vi "Panel.vi"() -> ()   [LabVIEW 2014]
uses:
  ISCO3.LLB/Pump start time.glb
  CONTROL.LLB/Remote/local.vi
panel:
  in  "btnExit":bool
  in  "?":bool
  out "TOTAL TIME, ms":u32
  in  "SAMPLE TIME, ms":u32=500
  out "Pump status.":T1(array[cluster])
  out "Multipump data.":T2 {"Total volume (liters)." format="%.5e"; "Pressure (psi)." format="%.5e"; "Flow rate (liters/min)." format="%.5e"}
  out "Digital input string.":string
  out "Analog input Voltages.":T3 {"ANLG5 = pin 2 , P107 auxiliary DB25 connector." format="%.2f"; "ANLG4 = analog input 1 of the accessory connector." format="%.2f"; "ANLG3 = analog input 2 of the accessory connector." format="%.2f"; "ANLG2 = pin 15 , P107 auxiliary DB25 connector and analog input 3 of the accessory connector." format="%.2f"; "ANLG1 = pin 21, P114." format="%.2f"}
  in  "Tasks.":T4
  in  "Remote/Local/External (0:Remote).":enum16{"REMOTE", "LOCAL", "EXTERNAL"}(ring)
  out "Pump C output.":T5={"Flow Rate A"=2.5, "FS Units A"=0, "Pressure A"=0.0, "PS Units A"=0, "Volume Remaining  C"=507.38, "Vol Units A"=0, "Status A"="STOPPED REMOTE  ", "Run time (Hr:Min:sec) A"=""} {"Vol Units A" items=["ml"]; "PS Units A" items=["psi", "atm", "bar", "kpa"]; "FS Units A" items=["ml/min", "ml/hr", "ul/min", "ul/hr"]; "Pressure A" format="%.2f"; "Flow Rate A" format="%.4f"; "Volume Remaining  C" scale=0.0..-1.0 scale format="%.1f"}
  out "Pump C Model":string="MODEL 500D PUMP; REV=G"
  in  "Pump C Settings":T6={"Mode A"=0, "Flow Setpoint A"=2.5, "FS Units A"=0, "Pressure Setpoint A"=100.0, "PS Units A"=0, "Refill Rate A"=204.0, "F=STOP/T=RUN"=FALSE} {"PS Units A" items=["psi", "atm", "bar", "kpa"]; "Refill Rate A" format="%.4f"; "Pressure Setpoint A" format="%.2f"; "FS Units A" items=["ml/min", "ml/hr", "ul/min", "ul/hr"]; "Flow Setpoint A" format="%.4f"; "Mode A" items=["Constant Flow", "Constant Pressure", "Refill", "Rapid Pressurization", "Single Pump Press Gradient", "Single Pump FR Gradient"]}
  out "Pump B output.":T7={"Flow Rate A"=15.0, "FS Units A"=0, "Pressure A"=0.0, "PS Units A"=0, "Volume Remaining  B"=94.65678, "Vol Units A"=0, "Status A"="STOPPED REMOTE  ", "Run time (Hr:Min:sec) A"=""} {"Vol Units A" items=["ml"]; "PS Units A" items=["psi", "atm", "bar", "kpa"]; "FS Units A" items=["ml/min", "ml/hr", "ul/min", "ul/hr"]; "Pressure A" format="%.2f"; "Flow Rate A" format="%.4f"; "Volume Remaining  B" scale format="%.1f"}
  out "Pump B Model":string="MODEL 100DM PUMP; REV=G"
  in  "Pump B Settings":T6={"Mode A"=0, "Flow Setpoint A"=15.0, "FS Units A"=0, "Pressure Setpoint A"=100.0, "PS Units A"=0, "Refill Rate A"=30.0, "F=STOP/T=RUN"=FALSE} {"PS Units A" items=["psi", "atm", "bar", "kpa"]; "Refill Rate A" format="%.4f"; "Pressure Setpoint A" format="%.2f"; "FS Units A" items=["ml/min", "ml/hr", "ul/min", "ul/hr"]; "Flow Setpoint A" format="%.4f"; "Mode A" items=["Constant Flow", "Constant Pressure", "Refill", "Rapid Pressurization", "Single Pump Press Gradient", "Single Pump FR Gradient"]}
  out "Pump A output.":T8={"Flow Rate A"=120.0, "FS Units A"=0, "Pressure A"=0.0, "PS Units A"=0, "Volume Remaining  A"=372.35144, "Vol Units A"=0, "Status A"="STOPPED REMOTE  ", "Run time (Hr:Min:sec) A"=""} {"Vol Units A" items=["ml"]; "PS Units A" items=["psi", "atm", "bar", "kpa"]; "FS Units A" items=["ml/min", "ml/hr", "ul/min", "ul/hr"]; "Pressure A" format="%.2f"; "Flow Rate A" format="%.4f"; "Volume Remaining  A" scale format="%.1f"}
  out "Pump A Model":string="MODEL 500D PUMP; REV=G"
  in  "Pump A Settings":T6={"Mode A"=0, "Flow Setpoint A"=120.0, "FS Units A"=0, "Pressure Setpoint A"=100.0, "PS Units A"=0, "Refill Rate A"=204.0, "F=STOP/T=RUN"=FALSE} {"PS Units A" items=["psi", "atm", "bar", "kpa"]; "Refill Rate A" format="%.4f"; "Pressure Setpoint A" format="%.2f"; "FS Units A" items=["ml/min", "ml/hr", "ul/min", "ul/hr"]; "Flow Setpoint A" format="%.4f"; "Mode A" items=["Constant Flow", "Constant Pressure", "Refill", "Rapid Pressurization", "Single Pump Press Gradient", "Single Pump FR Gradient"]}
  in  "Control mode (0:INDEPENDENT).":T9(ring)
  # "Status"
  # "Pump Model"
  # "Mode"
  # "Flow  Rate Setpt"
  # "Pressure Setpt"
  # "Refill Rate Setpt"
  # "STOP/RUN"
  # "C"
  # "Volume Remaining"
  # "Run Duration"
  # "B"
  # "Volume Remaining"
  # "Run Duration"
  # "A"
  # "Volume Remaining"
  # "Run Duration"
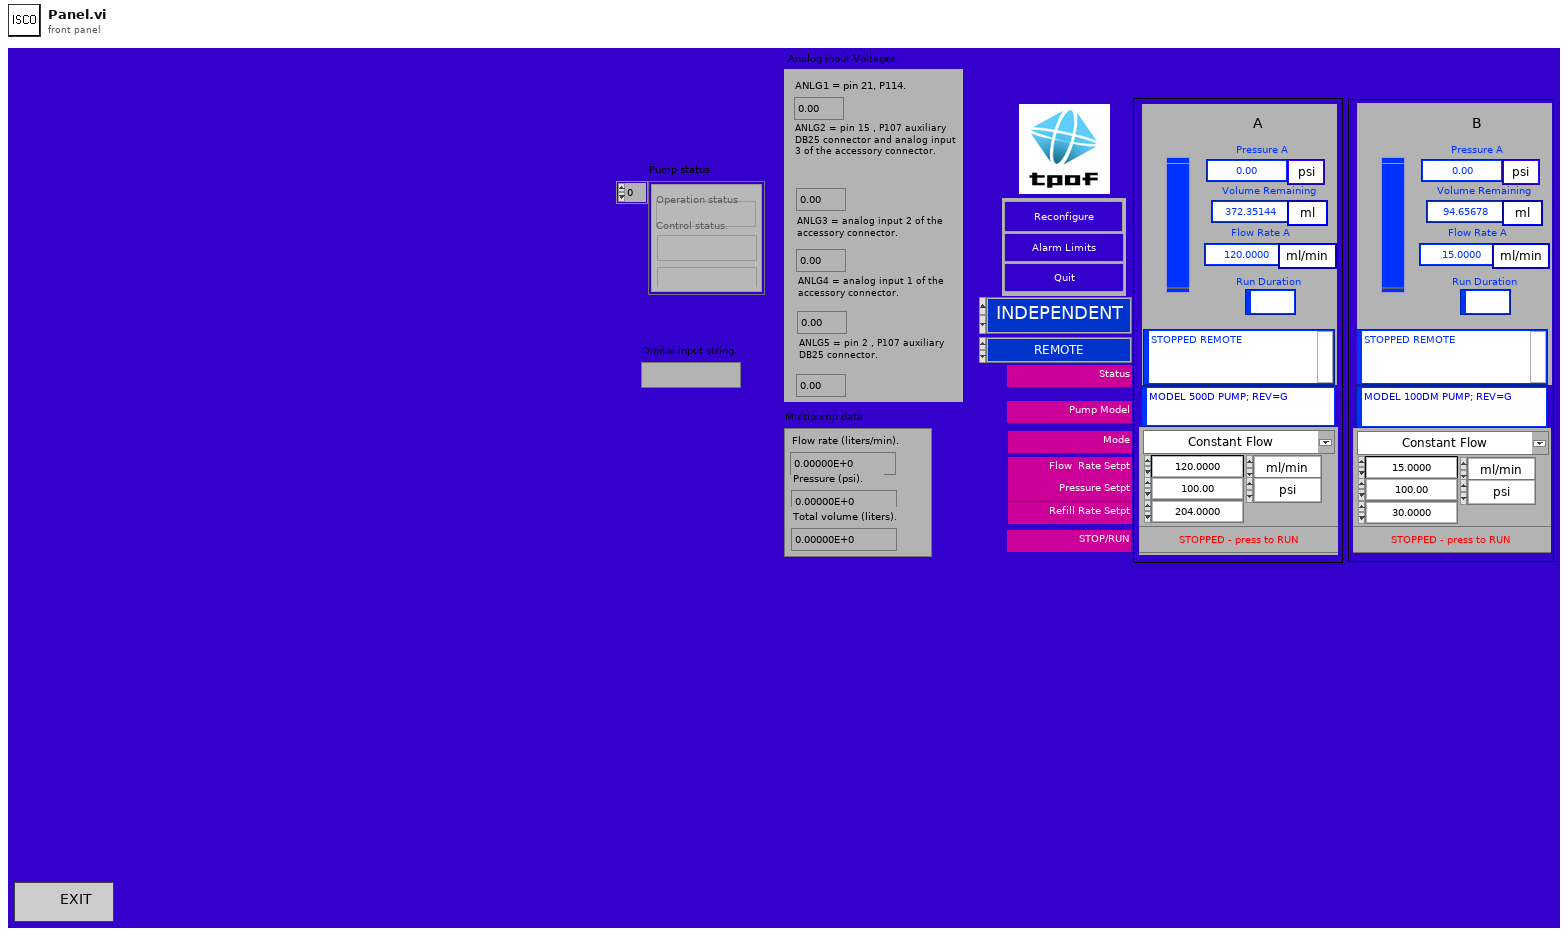
[diagram p1: front panel]
types:
  T1 = cluster{"Operation status":string, "Control status.  ":string, "Problem status.  ":string}[]
  T2 = cluster{"Flow rate (liters/min).  ":dbl, "Pressure (psi).  ":dbl, "Total volume (liters).  ":dbl}
  T3 = cluster{"ANLG1 = pin 21, P114.  ":dbl, "ANLG2 = pin 15 , P107 auxiliary DB25 connector and analog input 3 of the accessory connector.  ":dbl, "ANLG3 = analog input 2 of the accessory connector.  ":dbl, "ANLG4 = analog input 1 of the accessory connector.  ":dbl, "ANLG5 = pin 2 , P107 auxiliary DB25 connector.  ":dbl}
  T4 = cluster{"Reconfigure":bool, "Alarm Limits":bool, "Quit":bool}
  T5 = cluster{"Flow Rate A":sgl, "FS Units A":u16, "Pressure A":sgl, "PS Units A":u16, "Volume Remaining  C":sgl, "Vol Units A":u16, "Status A":string, "Run time (Hr:Min:sec) A":string}
  T6 = cluster{"Mode A":u16, "Flow Setpoint A":sgl, "FS Units A":u16, "Pressure Setpoint A":sgl, "PS Units A":u16, "Refill Rate A":sgl, "F=STOP/T=RUN":bool}
  T7 = cluster{"Flow Rate A":sgl, "FS Units A":u16, "Pressure A":sgl, "PS Units A":u16, "Volume Remaining  B":sgl, "Vol Units A":u16, "Status A":string, "Run time (Hr:Min:sec) A":string}
  T8 = cluster{"Flow Rate A":sgl, "FS Units A":u16, "Pressure A":sgl, "PS Units A":u16, "Volume Remaining  A":sgl, "Vol Units A":u16, "Status A":string, "Run time (Hr:Min:sec) A":string}
  T9 = enum16{"INDEPENDENT", "CONTIN CONST FLOW", "CONTIN CONST PRESS", "MODIFIER"}
  T10 = cluster{"Serial port":i32, "Baud rate":u16, "Controller":i32}
  T11 = cluster{"Mode A":u16, "Flow Setpoint A":sgl, "FS Units A":u16, "Pressure Setpoint A":sgl, "PS Units A":u16, "Refill Rate A":sgl, "F=STOP/T=RUN":bool}[]
  T12 = cluster{"Pump A.  ":string, "Pump B.  ":string, "Pump C.  ":string}
  T13 = cluster{"Maximum pressure (current units). ":sgl, "Maximum flow rate (current units).  ":sgl, "Maximum refill rate (currents units).  ":sgl, "Maximum volume (milliliters).  ":sgl}
  T14 = cluster{"Maximum pressure ":sgl, "Maximum flow rate.  ":sgl, "Maximum refill rate.  ":sgl, "Maximum volume.  ":sgl}
  T15 = cluster{"Maximum pressure setpoint.  ":sgl, "Minimum pressure setpoint":sgl, "Maximum flow rate.  ":sgl, "Minimum flow rate.  ":sgl, "Maximum flow rate in constant pressure mode.  ":sgl}
  T16 = cluster{"Maximum pressure setpoint (psi).  ":sgl, "Minimum pressure setpoint (psi).  ":sgl, "Maximum flow rate (liters/minute).  ":sgl, "Minimum flow rate (liters/minute).  ":sgl, "Maximum flow rate in constant pressure mode (liters/minute).  ":sgl}
  T17 = cluster{cluster{"Maximum pressure ":sgl, "Maximum flow rate.  ":sgl, "Maximum refill rate.  ":sgl, "Maximum volume.  ":sgl}[], cluster{"Maximum pressure setpoint (psi).  ":sgl, "Minimum pressure setpoint (psi).  ":sgl, "Maximum flow rate (liters/minute).  ":sgl, "Minimum flow rate (liters/minute).  ":sgl, "Maximum flow rate in constant pressure mode (liters/minute).  ":sgl}[]}
  T18 = enum32{"No op", "Reconfigure", "alarm limits", "Quit"}
  T19 = cluster{"Duration of run - pump A\n(Hours:minutes:seconds":string, "Duration of run - pump B\n(Hours:minutes:seconds":string, "Duration of run - pump C\n(Hours:minutes:seconds":string}
  T20 = cluster{"Time limit exceeded?  ":bool, "Bad checksum?":bool, "Busy?":bool}
  T21 = cluster{"Flow rate.  ":sgl, "Pressure.  ":sgl, "Volume remaining.  ":sgl, "Operation status.  ":string, "Control status.  ":string, "Problem status.  ":string}[]
  T22 = cluster{"ANLG1 = pin 21, P114.  ":dbl, "ANLG2 = pin 15 , P107 auxiliary DB25 connector and analog input 2 of the accessory connector.  ":dbl, "ANLG3 = analog input 2 of the accessory connector.  ":dbl, "ANLG4 = analog input 1 of the accessory connector.  ":dbl, "ANLG5 = pin 2 , P107 auxiliary DB25 connector.  ":dbl}
  T23 = cluster{"Maximum pressure setpoint (psi).  ":sgl, "Minimum pressure setpoint (psi).  ":sgl, "Maximum flow rate (liters/minute).  ":sgl, "Minimum flow rate (liters/minute).  ":sgl, "Maximum flow rate in constant pressure mode (liters/minute).  ":sgl}[]
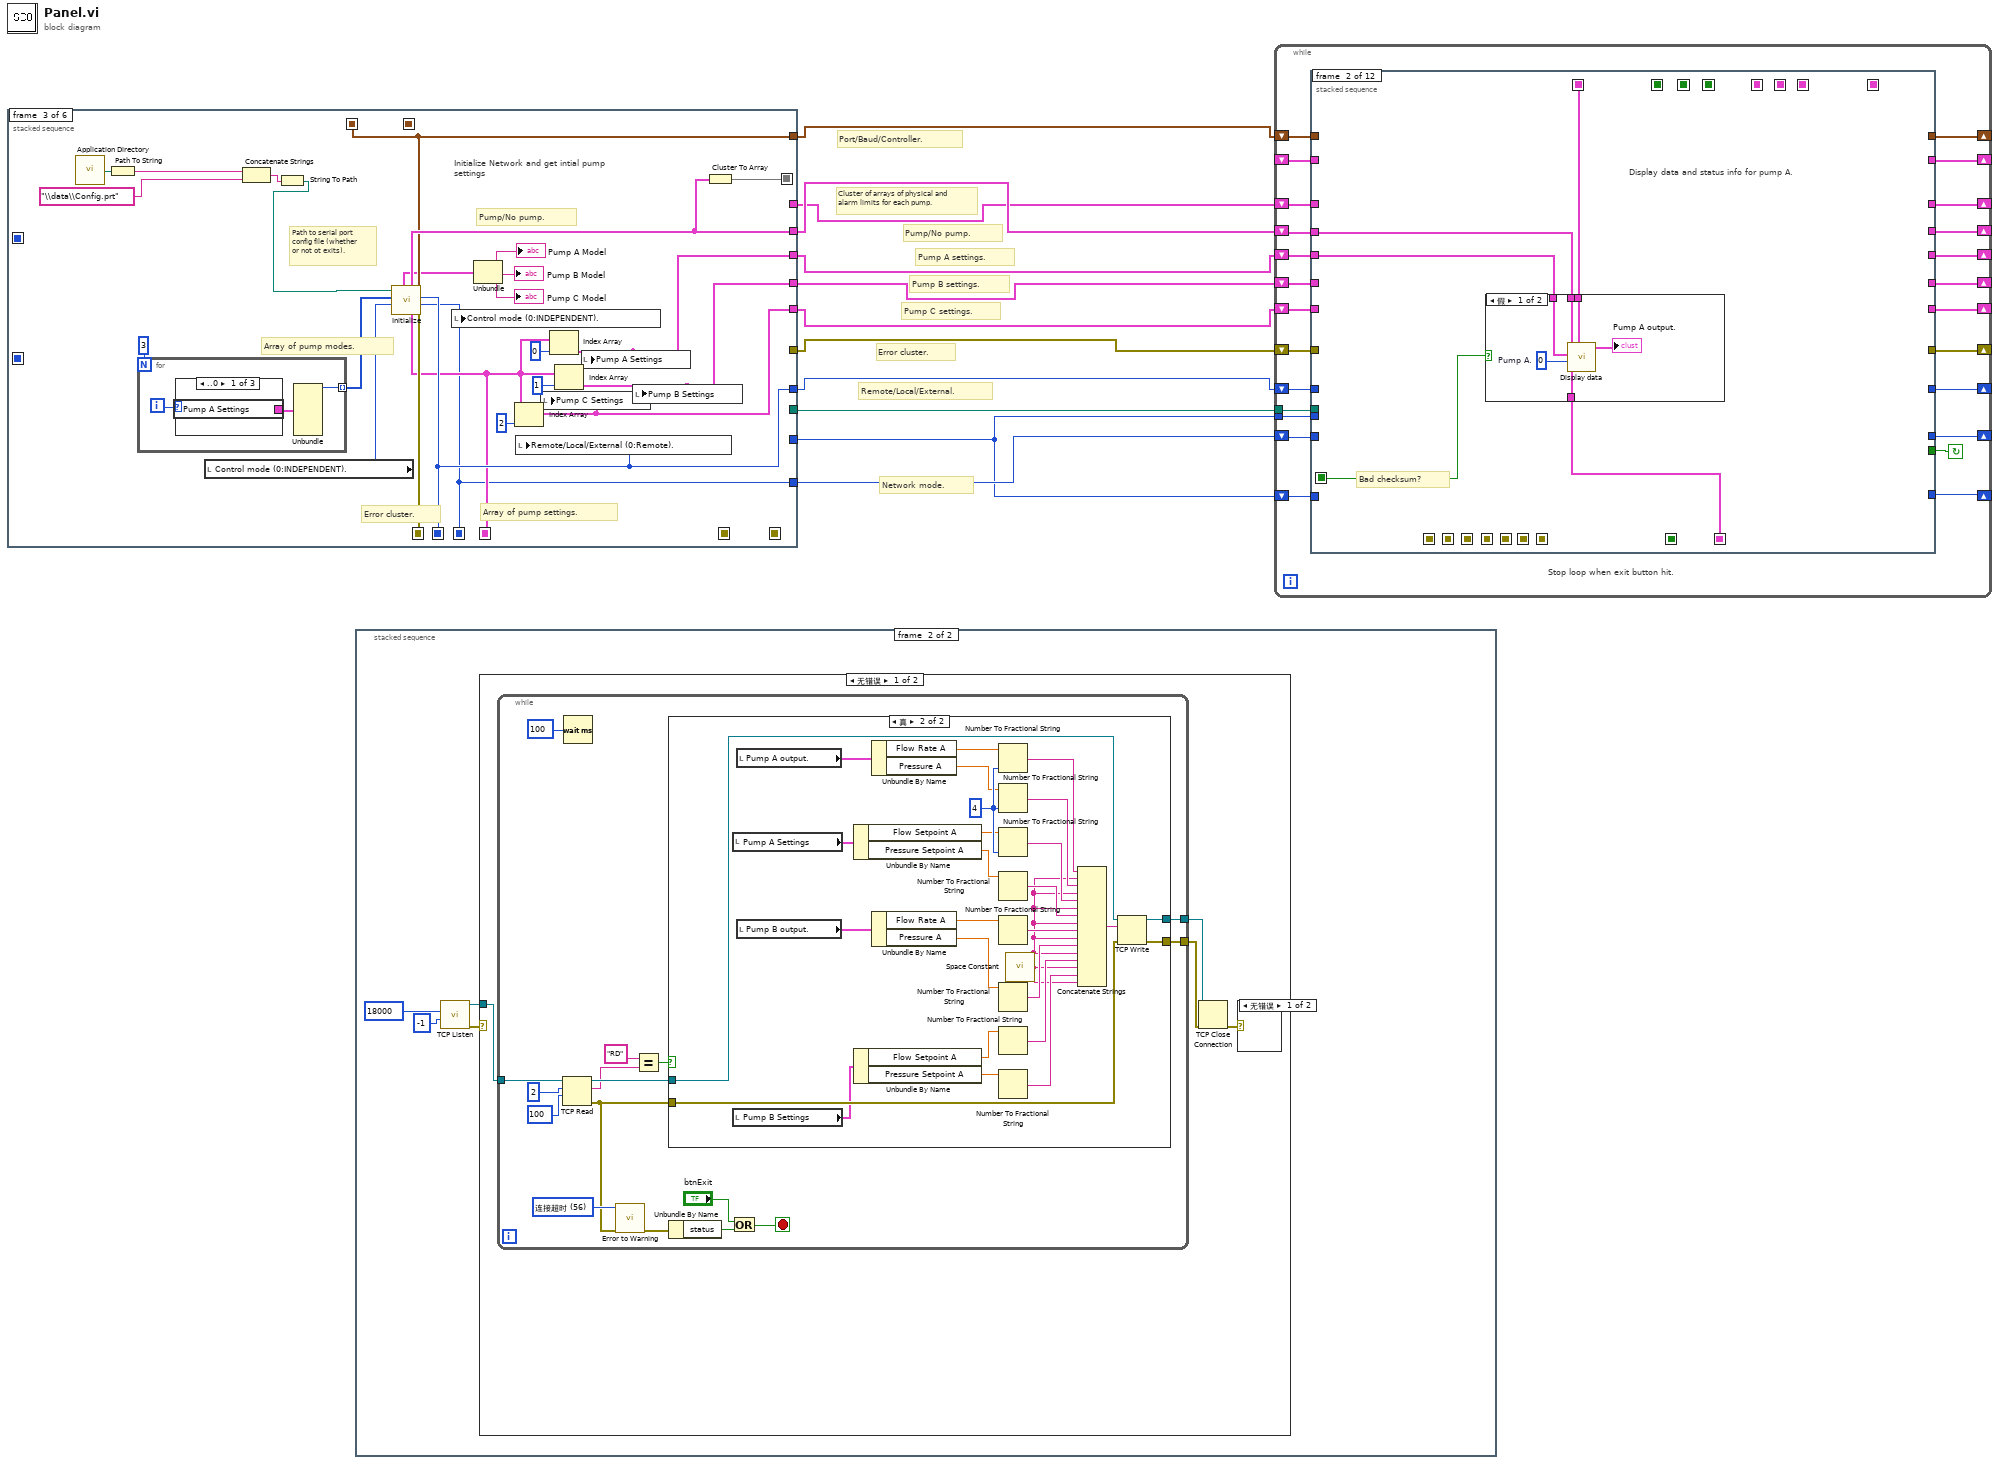
[diagram p0: block diagram]
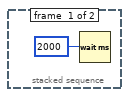
[diagram p2: hidden frame]
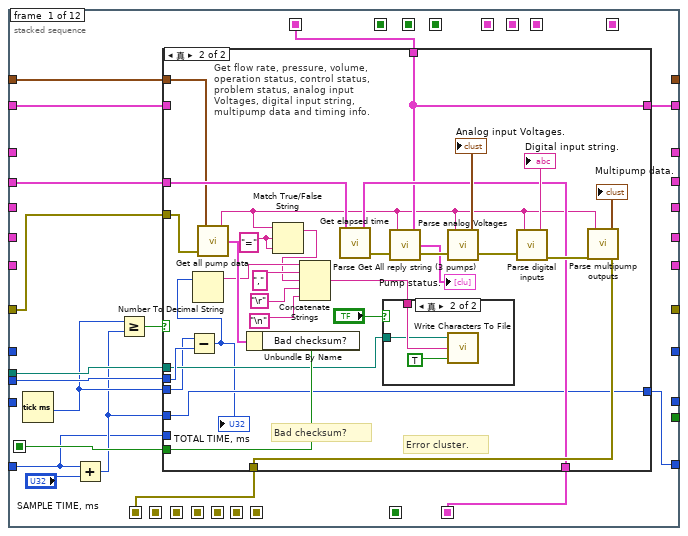
[diagram p6: hidden frame]
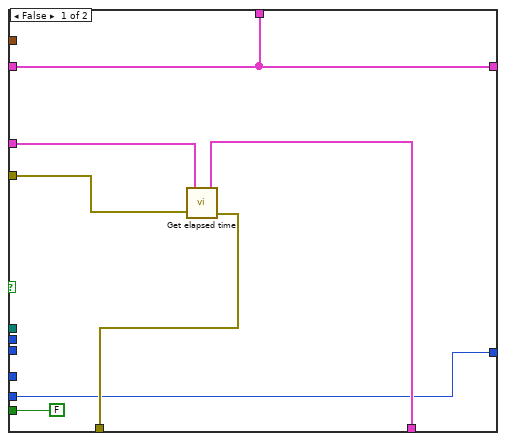
[diagram p7: hidden frame]
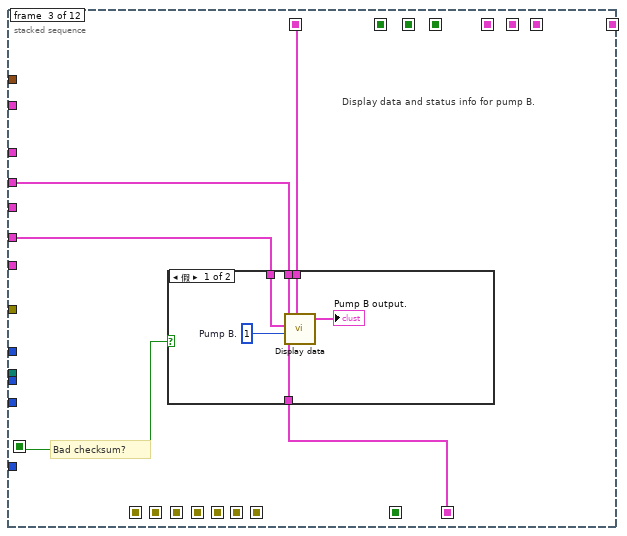
[diagram p10: hidden frame]
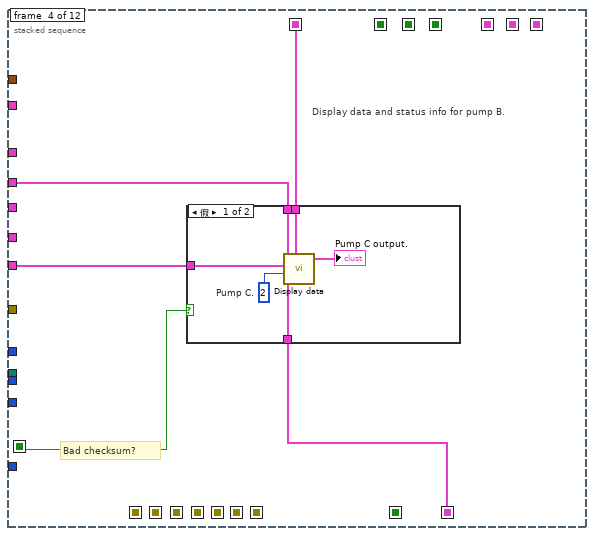
[diagram p12: hidden frame]
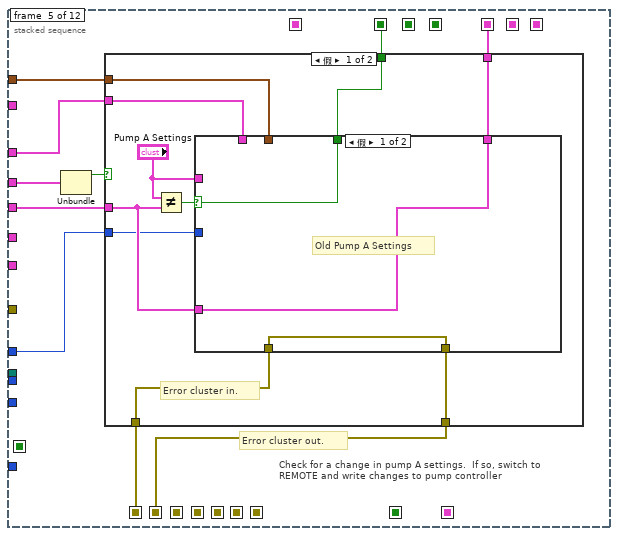
[diagram p14: hidden frame]
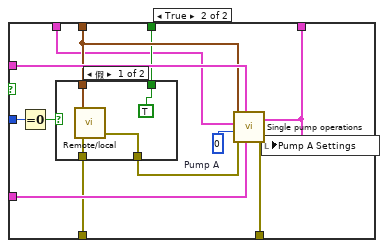
[diagram p15: hidden frame]
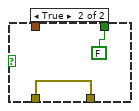
[diagram p16: hidden frame]
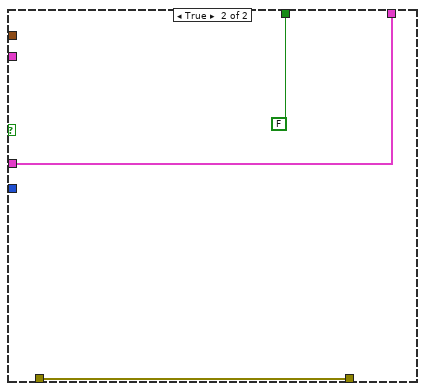
[diagram p17: hidden frame]
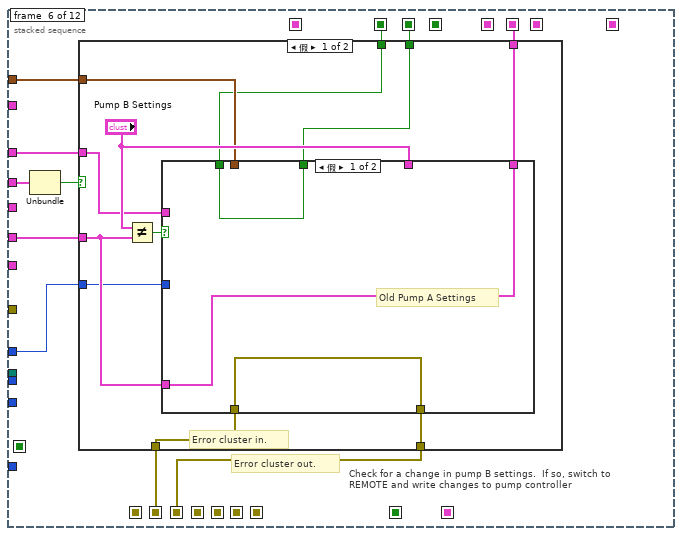
[diagram p18: hidden frame]
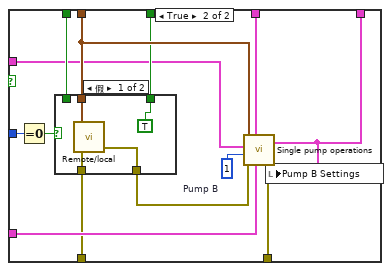
[diagram p19: hidden frame]
diagram:
  # "Cluster of arrays of physical and alarm limits for each pump."
  # "Network mode."
  # "Pump C settings."
  # "Pump B settings."
  # "Pump A settings."
  # "Remote/Local/External."
  # "Port/Baud/Controller."
  # "Error cluster."
  # "Pump/No pump."
  n1 = stacked-sequence {
    seq-local: [_ _ w40 _ _ _] -> [_ _ _ w56 w142 w215]
    seq-local: [_ _ w36 _ _ _] -> [_ _ _ w54 w137 w219]
    seq-local: [_ _ w39 _ _ _] -> [_ _ _ w53 _ _]
    seq-local: [_ _ w26 _ _ _] -> [_ _ _ _ _ w216]
    seq-local: [_ _ _ w55 _ _] -> [_ _ _ _ w138 _]
    seq-local: [_ _ w25 _ _ _] -> [_ _ _ _ _ w214]
    seq-local: [_ _ w23 _ _ _] -> [_ _ _ _ _ w213]
    seq-local: [_ _ _ w51 _ _] -> [_ _ _ _ w140 _]
    seq-local: [_ _ _ w50 _ _] -> [_ _ _ _ w139 _]
    seq-local: [_ _ _ _ w141 _] -> [_ _ _ _ _ w212]
    seq-local: [_ _ _ w49 _ _] -> [_ _ _ _ w136 _]
    tunnel: [_ _ w37 _ _ _] -> w9
    tunnel: [_ _ _ _ _ w218] -> w11
    tunnel: [_ _ w36 _ _ _] -> w10
    tunnel: [_ _ w26 _ _ _] -> w8
    tunnel: [_ _ w27 _ _ _] -> w7
    tunnel: [_ _ w28 _ _ _] -> w6
    tunnel: [_ _ w29 _ _ _] -> w5
    tunnel: [_ _ w23 _ _ _] -> w4
    tunnel: [_ _ _ _ w134 _] -> w3
    tunnel: [_ w13 _ _ _ _] -> w2
    tunnel: [_ _ _ _ _ w211] -> w1
    frame #0 {
      w12 = -1
      # "Initialize timing global variables"
      n2 = global write "Pump start time.glb" "Pump A start time (milliseconds)."(w12) -> ()
      n3 = global write "Pump start time.glb" "Pump B start time (milliseconds)."(w12) -> ()
      n4 = global write "Pump start time.glb" "Pump C start time (milliseconds)."(w12) -> ()
    }
    frame #1 {
      n5 = call <vilib>:"Application Directory.vi"() -> ("Application Directory"=w16:path)
      n6 = Path To String(path=w16) -> (string=w15:string)
      n7 = Concatenate Strings(w15, "\\data\\DATA.CSV" ("字符串")) -> (w17:string)
      n8 = String To Path(string=w17) -> (path=w13:path)
    }
    frame #2 {
      # "Array of pump settings."
      # "Array of pump modes."
      # "Path to serial port config file (whether or not ot exits)."
      # "Error cluster."
      # "Pump/No pump."
      # "Initialize Network and get intial pump settings"
      n9 = call <vilib>:"Application Directory.vi"() -> ("Application Directory"=w21:path)
      n10 = Path To String(path=w21) -> (string=w20:string)
      n11 = for {
        N: 3 -> [_]
        tunnel: [w43] -> w34 mode=indexing
        i -> [w44]
        n12 = case shown="..0" w44 {
          tunnel: [w46 w47 w48] -> w45
          frame ..0 {
            n13 = local read "Pump A Settings"() -> (w46:T6)
          }
          frame 1 {
            n14 = local read "Pump B Settings"() -> (w47:T6)
          }
          frame 2.. {
            n15 = local read "Pump C Settings"() -> (w48:T6)
          }
        }
        n16 = Unbundle(w45) -> ("Mode A"=w43:u16)  [unwired: 6 out]
      }
      n17 = local read "Control mode (0:INDEPENDENT)."() -> (w33:T9)
      n18 = Concatenate Strings(w20, "\\data\\Config.prt" ("字符串")) -> (w22:string)
      n19 = String To Path(string=w22) -> (path=w18:path)
      n20 = call "Initialize.vi"("Mode (0:INDEPENDENT)."=w33, "Pump Mode"=w34, "Serial port config file (empty)."=w18) -> ("Error out."=w39:errorcluster, "Mode (0:INDEPENDENT)."=w23:T9, "Remote/Local/External (0:Remote)."=w26:enum16{"REMOTE", "LOCAL", "EXTERNAL"}, "Port/Baud/Controller"=w36:T10, "Array of pump settings."=w25:T11, "Pump? (F:pump present)."=w37:cluster{bool, bool, bool}, "Pump model info."=w24:T12)  [unwired: 2 in]
      n21 = local write "Control mode (0:INDEPENDENT)."(w23) -> ()
      n22 = Unbundle(w24) -> ("Pump A."=→"Pump A Model":string, "Pump B."=→"Pump B Model":string, "Pump C."=→"Pump C Model":string)
      n23 = Index Array(array=w25, index=2) -> (element=w27:T6)
      n24 = local write "Remote/Local/External (0:Remote)."(w26) -> ()
      n25 = local write "Pump C Settings"(w27) -> ()
      n26 = Index Array(array=w25, index=0) -> (element=w29:T6)
      n27 = Index Array(array=w25, index=1) -> (element=w28:T6)
      n28 = local write "Pump A Settings"(w29) -> ()
      n29 = local write "Pump B Settings"(w28) -> ()
      n30 = Cluster To Array(cluster=w37) -> (array=w40:bool[])
    }
    frame #3 {
      # "Scale the volume remaining graphics and get physical limits."
      # "Port/Baud/Controller."
      # "Error cluster."
      # "Error cluster."
      # "Pump/No pump."
      n31 = call "Get units.vi"("Port/Baud/Controller"=w54, "Error in (no error)."=w53) -> ("Flow rate units."=w51:enum16{"ML/MIN", "ML/HR", "UL/MIN", "UL/HR"}, "Pressure units."=w50:enum16{"PSI", "ATM", "BAR", "KPa"}, "Error out."=w52:errorcluster)
      n32 = for {
        tunnel: w56 -> [w63] mode=indexing
        shift-right: [w61] -> w55
        shift-left: w52 -> [w62]
        tunnel: w54 -> [w60]
        tunnel: w51 -> [w59]
        tunnel: w50 -> [w58]
        tunnel: [w57] -> w49 mode=indexing
        i -> [w64]
        n33 = case shown="..0" w64 {
          selector: w64 -> [w71 w94 w117]
          tunnel: w63 -> [w72 w95 w118]
          tunnel: w62 -> [w70 w93 w116]
          tunnel: [w69 w92 w115] -> w61
          tunnel: w60 -> [w68 w91 w114]
          tunnel: w59 -> [w67 w90 w113]
          tunnel: w58 -> [w66 w89 w112]
          tunnel: [w65 w88 w111] -> w57
          frame ..0 {
            n34 = case shown="真" w72 {
              tunnel: w71 -> [w81 _]
              tunnel: w70 -> [w80 w87]
              tunnel: [w74 w87] -> w69
              tunnel: w68 -> [w79 _]
              tunnel: w67 -> [w78 _]
              tunnel: w66 -> [w77 _]
              tunnel: [w73 w86] -> w65
              frame False {
                n35 = call "Get range.vi"("Error in (no error)."=w80, "Pump (0:A)."=w81, "Port/Baud/Controller"=w79) -> ("Error out."=w75:errorcluster, "Physical pump limits."=w76:T13)  [unwired: 1 in]
                n36 = call "Range to standard units.vi"("Error in (no error)."=w75, "Physical limits (current units)."=w76, "Current pressure Units (0:psi)"=w77, "Current flow rate Units (0:ml/min)"=w78) -> ("Error out."=w74:errorcluster, "Physical limits (psi and ml/min)."=w73:T14)
                n37 = Unbundle By Name(w76) -> ("Maximum volume (milliliters)."=w82:sgl)
                n38 = To Double Precision Float(number=w82) -> (double precision float=w84:dbl)
                n39 = property on="Volume Remaining  A" class="Slide (严格)"("Scale.Range:Minimum"=0.0, "Scale.Range:Maximum"=w84) -> ()  [unwired: 2 in, 2 out]
              }
              frame True {
                w85 = sgl 0.0
                n40 = Bundle(w85, w85, w85, w85) -> (w86:cluster{sgl, sgl, sgl, sgl})  [unwired: 1 in]
              }
            }
          }
          frame 1 {
            n41 = case shown="假" w95 {
              tunnel: w94 -> [w106 _]
              tunnel: w93 -> [w105 w110]
              tunnel: [w99 w110] -> w92
              tunnel: w91 -> [w104 _]
              tunnel: w90 -> [w103 _]
              tunnel: w89 -> [w102 _]
              tunnel: [w96 w108] -> w88
              frame False {
                n42 = call "Get range.vi"("Error in (no error)."=w105, "Pump (0:A)."=w106, "Port/Baud/Controller"=w104) -> ("Error out."=w100:errorcluster, "Physical pump limits."=w101:T13)  [unwired: 1 in]
                n43 = call "Range to standard units.vi"("Error in (no error)."=w100, "Physical limits (current units)."=w101, "Current pressure Units (0:psi)"=w102, "Current flow rate Units (0:ml/min)"=w103) -> ("Error out."=w99:errorcluster, "Physical limits (psi and ml/min)."=w96:T14)
                n44 = Unbundle By Name(w101) -> ("Maximum volume (milliliters)."=w107:sgl)
                n45 = To Double Precision Float(number=w107) -> (double precision float=w98:dbl)
                n46 = property on="Volume Remaining  B" class="Slide (严格)"("Scale.Range:Minimum"=0.0, "Scale.Range:Maximum"=w98) -> ()  [unwired: 2 in, 2 out]
              }
              frame True {
                w109 = sgl 0.0
                n47 = Bundle(w109, w109, w109, w109) -> (w108:cluster{sgl, sgl, sgl, sgl})  [unwired: 1 in]
              }
            }
          }
          frame 2.. {
            n48 = case shown="假" w118 {
              tunnel: w117 -> [w129 _]
              tunnel: w116 -> [w128 w133]
              tunnel: [w122 w133] -> w115
              tunnel: w114 -> [w127 _]
              tunnel: w113 -> [w126 _]
              tunnel: w112 -> [w125 _]
              tunnel: [w119 w131] -> w111
              frame False {
                n49 = call "Get range.vi"("Error in (no error)."=w128, "Pump (0:A)."=w129, "Port/Baud/Controller"=w127) -> ("Error out."=w123:errorcluster, "Physical pump limits."=w124:T13)  [unwired: 1 in]
                n50 = call "Range to standard units.vi"("Error in (no error)."=w123, "Physical limits (current units)."=w124, "Current pressure Units (0:psi)"=w125, "Current flow rate Units (0:ml/min)"=w126) -> ("Error out."=w122:errorcluster, "Physical limits (psi and ml/min)."=w119:T14)
                n51 = Unbundle By Name(w124) -> ("Maximum volume (milliliters)."=w130:sgl)
                n52 = To Double Precision Float(number=w130) -> (double precision float=w120:dbl)
                n53 = property on="Volume Remaining  C" class="Slide (严格)"("Scale.Range:Minimum"=0.0, "Scale.Range:Maximum"=w120) -> ()  [unwired: 2 in, 2 out]
              }
              frame True {
                w132 = sgl 0.0
                n54 = Bundle(w132, w132, w132, w132) -> (w131:cluster{sgl, sgl, sgl, sgl})  [unwired: 1 in]
              }
            }
          }
        }
      }
    }
    frame #4 {
      # "Port/Baud/Controller."
      # "Error cluster."
      # "Error cluster."
      # "Get alarm limits."
      # "Pump/No pump."
      n55 = for {
        tunnel: w142 -> [w149] mode=indexing
        shift-right: [w147] -> w141
        shift-left: w138 -> [w148]
        tunnel: w137 -> [w146]
        tunnel: w140 -> [w145]
        tunnel: w139 -> [w144]
        tunnel: [w143] -> w135 mode=indexing
        i -> [w150]
        n56 = case shown="2.." w150 {
          selector: w150 -> [w157 w177 w197]
          tunnel: w149 -> [w158 w178 w198]
          tunnel: w148 -> [w156 w176 w196]
          tunnel: [w155 w175 w195] -> w147
          tunnel: w146 -> [w154 w174 w194]
          tunnel: w145 -> [w153 w173 w193]
          tunnel: w144 -> [w152 w172 w192]
          tunnel: [w151 w171 w191] -> w143
          frame ..0 {
            n57 = case shown="假" w158 {
              tunnel: w157 -> [w167 _]
              tunnel: w156 -> [w166 w170]
              tunnel: [w161 w170] -> w155
              tunnel: w154 -> [w165 _]
              tunnel: w153 -> [w164 _]
              tunnel: w152 -> [w163 _]
              tunnel: [w160 w169] -> w151
              frame False {
                n58 = call "Get alarm limit setpoints.vi"("Error in (no error)."=w166, "Pump (0:A)."=w167, "Port/Baud/Controller"=w165) -> ("Error out."=w162:errorcluster, "Alarm limits setpoints (in the currently selected units)."=w159:T15)  [unwired: 1 in]
                n59 = call "AL units to standard units.vi"("Error in (no error)."=w162, "Alarm limits setpoint (in current units)."=w159, "Pressure Units (0:psi)"=w163, "Flow rate Units (0:ml/min)"=w164) -> ("Error out."=w161:errorcluster, "Alarm limits setpoints (in standard units)."=w160:T16)
              }
              frame True {
                w168 = sgl 0.0
                n60 = Bundle(w168, w168, w168, w168, w168) -> (w169:cluster{sgl, sgl, sgl, sgl, sgl})  [unwired: 1 in]
              }
            }
          }
          frame 1 {
            n61 = case shown="假" w178 {
              tunnel: w177 -> [w187 _]
              tunnel: w176 -> [w186 w190]
              tunnel: [w181 w190] -> w175
              tunnel: w174 -> [w185 _]
              tunnel: w173 -> [w184 _]
              tunnel: w172 -> [w183 _]
              tunnel: [w180 w189] -> w171
              frame False {
                n62 = call "Get alarm limit setpoints.vi"("Error in (no error)."=w186, "Pump (0:A)."=w187, "Port/Baud/Controller"=w185) -> ("Error out."=w182:errorcluster, "Alarm limits setpoints (in the currently selected units)."=w179:T15)  [unwired: 1 in]
                n63 = call "AL units to standard units.vi"("Error in (no error)."=w182, "Alarm limits setpoint (in current units)."=w179, "Pressure Units (0:psi)"=w183, "Flow rate Units (0:ml/min)"=w184) -> ("Error out."=w181:errorcluster, "Alarm limits setpoints (in standard units)."=w180:T16)
              }
              frame True {
                w188 = sgl 0.0
                n64 = Bundle(w188, w188, w188, w188, w188) -> (w189:cluster{sgl, sgl, sgl, sgl, sgl})  [unwired: 1 in]
              }
            }
          }
          frame 2.. {
            n65 = case shown="假" w198 {
              tunnel: w197 -> [w207 _]
              tunnel: w196 -> [w206 w210]
              tunnel: [w201 w210] -> w195
              tunnel: w194 -> [w205 _]
              tunnel: w193 -> [w204 _]
              tunnel: w192 -> [w203 _]
              tunnel: [w200 w209] -> w191
              frame False {
                n66 = call "Get alarm limit setpoints.vi"("Error in (no error)."=w206, "Pump (0:A)."=w207, "Port/Baud/Controller"=w205) -> ("Error out."=w202:errorcluster, "Alarm limits setpoints (in the currently selected units)."=w199:T15)  [unwired: 1 in]
                n67 = call "AL units to standard units.vi"("Error in (no error)."=w202, "Alarm limits setpoint (in current units)."=w199, "Pressure Units (0:psi)"=w203, "Flow rate Units (0:ml/min)"=w204) -> ("Error out."=w201:errorcluster, "Alarm limits setpoints (in standard units)."=w200:T16)
              }
              frame True {
                w208 = sgl 0.0
                n68 = Bundle(w208, w208, w208, w208, w208) -> (w209:cluster{sgl, sgl, sgl, sgl, sgl})  [unwired: 1 in]
              }
            }
          }
        }
      }
      n69 = Bundle(w136, w135) -> (w134:T17)  [unwired: 1 in]
    }
    frame #5 {
      # "Network mode."
      # "Array of pump settings."
      # "Port/Baud/Controller."
      # "Pump/No pump."
      # "Error cluster."
      # "If in remote mode set the pump operation mode"
      n70 = Equal To 0?(x=w216) -> (x = 0?=w217:bool)
      n71 = case shown="真" w217 {
        tunnel: w212 -> [w220 w226]
        tunnel: [w220 w222] -> w218
        tunnel: w219 -> [_ w224]
        tunnel: w215 -> [_ w227]
        tunnel: w214 -> [_ w223]
        tunnel: w213 -> [_ w221]
        frame False {
        }
        frame True {
          n72 = for {
            tunnel: w227 -> [w234] mode=indexing
            shift-right: [w230] -> w225
            shift-left: w226 -> [w232]
            tunnel: w224 -> [w233]
            tunnel: w223 -> [w228] mode=indexing
            i -> [w231]
            n73 = Unbundle(w228) -> ("Mode A"=w229:u16)  [unwired: 6 out]
            n74 = case shown="假" w234 {
              tunnel: w233 -> [w239 _]
              tunnel: w232 -> [w238 w240]
              tunnel: w231 -> [w237 _]
              tunnel: [w236 w240] -> w230
              tunnel: w229 -> [w235 _]
              frame False {
                n75 = call "Set pump mode.vi"("Error in (no error)."=w238, "Mode (0:const flow)."=w235, "Pump (0:A)."=w237, "Port/Baud/Controller"=w239) -> ("Error out."=w236:errorcluster)  [unwired: 2 in]
              }
              frame True {
              }
            }
          }
          n76 = call "Set controller mode.vi"("Error in (no error)."=w225, "Mode (0:INDEPENDENT)."=w221, "Port/Baud/Controller"=w224) -> ("Error out."=w222:errorcluster)  [unwired: 2 in]
        }
      }
      n77 = Tick Count (ms)() -> (millisecond timer value=w211:u32)
    }
  }
  n78 = stacked-sequence {
    frame #0 {
      n79 = Wait (ms)(milliseconds to wait=u32 2000 ("等待时间（毫秒）")) -> ()  [unwired: 1 out]
    }
    frame #1 {
      n80 = call <vilib>:"TCP Listen.vi"("timeout ms (wait forever: -1)"=-1, "port"=u16 18000) -> ("error out"=w243:errorcluster, "connection ID"=w242:refnum<k5>)  [unwired: 5 in, 3 out]
      n81 = case shown="无错误" w243 {
        tunnel: w242 -> [w249 _]
        frame No Error {
          n82 = while {
            tunnel: w249 -> [w265]
            tunnel: [w255] -> w248
            tunnel: [w254] -> w247
            stop <- w250 stop-if-true
            w262 = 56 items=["无错误", "参数错误", "内存已满", "超出区域", "文件结束", "文件已打开", "一般文件IO错误", "未找到文件", "文件权限错误", "磁盘已满", "路径副本", "打开过多文件", "未启用", "未找到资源文件", "无法添加资源", "未找到资源", "未找到图像", "图像内存错误", "画笔不存在", "配置错误类型", "配置未找到解析段", "配置解析错误", "配置内存错误", "错误外部代码格式", "错误外部代码偏移量", "外部代码不存在", "空窗口", "销毁窗口错误", "空菜单", "打印已中止", "错误打印记录", "打印驱动程序错误", "打印时窗口错误", "打印时内存错误", "打印对话框错误", "一般打印错误", "无效设备引用句柄", "设备未找到", "设备参数错误", "设备单位错误", "无法打开设备", "设备调用已中止", "一般错误", "用户已取消", "对象ID过低", "对象ID过高", "对象不在堆中", "未知的堆", "错误DefProc ID", "DefProc不在表格中", "范围外信息", "空方法", "未知信息", "不支持管理器调用", "错误地址", "连接过程中", "连接超时", "连接过程中", "不支持网络属性", "网络错误", "正在使用的地址", "系统缺少内存", "连接已中止", "连接已拒绝", "连接未建立", "连接已建立", "连接已关闭", "初始化错误（交互应用程序管理器）", "错误事件发生", "等待无约束事件发生处理程序", "事件发生队列溢出", "错误路径", "未发出信号量", "未识别类型（交互应用程序管理器）"] ("1st Error to Convert")
            n83 = TCP Read(connection ID=w265, bytes to read=2 ("读取的字节"), 9:100 ("超时毫秒(25000)")) -> (connection ID out=w260:refnum<k5>, data out=w258:string, error out=w253:errorcluster)  [unwired: 2 in]
            n84 = Wait (ms)(milliseconds to wait=u32 100 ("等待时间（毫秒）")) -> ()  [unwired: 1 out]
            n85 = call <vilib>:"Error to Warning.vi"("1st Error to Convert"=w262, "error in"=w253) -> ("warning out"=w261:errorcluster)  [unwired: 13 in]
            n86 = Equal?(x="RD" ("真字符串"), y=w258) -> (x = y?=w257:bool)
            n87 = case shown="真" w257 {
              tunnel: w260 -> [w267 w294]
              tunnel: [w267 w291] -> w255
              tunnel: [w266 w290] -> w254
              tunnel: w253 -> [w266 w289]
              frame False {
              }
              frame True {
                w287 = i16 4 ("精度(6)")
                n88 = local read "Pump A Settings"() -> (w282:T6)
                n89 = local read "Pump B Settings"() -> (w273:T6)
                n90 = local read "Pump A output."() -> (w285:T8)
                n91 = local read "Pump B output."() -> (w278:T7)
                n92 = Unbundle By Name(w282) -> ("Flow Setpoint A"=w281:sgl, "Pressure Setpoint A"=w279:sgl)
                n93 = Unbundle By Name(w273) -> ("Flow Setpoint A"=w272:sgl, "Pressure Setpoint A"=w270:sgl)
                n94 = Unbundle By Name(w285) -> ("Flow Rate A"=w284:sgl, "Pressure A"=w283:sgl)
                n95 = Unbundle By Name(w278) -> ("Flow Rate A"=w277:sgl, "Pressure A"=w275:sgl)
                n96 = Number To Fractional String(number=w284, precision (6)=w287) -> (F-format string=w293:string)  [unwired: 2 in]
                n97 = Number To Fractional String(number=w283, precision (6)=w287) -> (F-format string=w288:string)  [unwired: 2 in]
                n98 = Number To Fractional String(number=w281, precision (6)=w287) -> (F-format string=w286:string)  [unwired: 2 in]
                n99 = Number To Fractional String(number=w279) -> (F-format string=w280:string)  [unwired: 3 in]
                n100 = Number To Fractional String(number=w277) -> (F-format string=w276:string)  [unwired: 3 in]
                n101 = Number To Fractional String(number=w275) -> (F-format string=w274:string)  [unwired: 3 in]
                n102 = Number To Fractional String(number=w272) -> (F-format string=w271:string)  [unwired: 3 in]
                n103 = Number To Fractional String(number=w270) -> (F-format string=w269:string)  [unwired: 3 in]
                n104 = call <vilib>:"Space Constant.vi"() -> ("String"=w268:string)
                n105 = Concatenate Strings(w293, w268, w288, w268, w286, w268, w280, w268, w276, w268, w274, w268, w271, w268, w269, w268) -> (w292:string)
                n106 = TCP Write(connection ID=w294, data in=w292, error in (no error)=w289) -> (connection ID out=w291:refnum<k5>, error out=w290:errorcluster)  [unwired: 1 in, 1 out]
              }
            }
            n107 = Unbundle By Name(w261) -> ("status"=w251:bool)
            n108 = Or(x="btnExit", y=w251) -> (x .or. y?=w250:bool)
          }
          n109 = TCP Close Connection(connection ID=w248, error in (no error)=w247) -> (error out=w246:errorcluster)  [unwired: 1 in, 1 out]
          n110 = case shown="无错误" w246 {
            frame No Error {
            }
            frame Error {
            }
          }
        }
        frame Error {
        }
      }
    }
  }
  n111 = while {
    tunnel: w1 -> [w295]
    tunnel: w2 -> [w296]
    shift-left: _ -> [w297]
    shift-right: [w298] -> _
    shift-left: w1 -> [w300]
    shift-right: [w299] -> _
    shift-left: w3 -> [w302]
    shift-right: [w301] -> _
    shift-left: w4 -> [w304]
    shift-right: [w303] -> _
    shift-left: w9 -> [w306]
    shift-right: [w305] -> _
    shift-left: w8 -> [w308]
    shift-right: [w307] -> _
    shift-left: w11 -> [w311]
    shift-right: [w310] -> _
    shift-left: w7 -> [w316]
    shift-right: [w315] -> _
    shift-left: w6 -> [w317]
    shift-right: [w309] -> _
    shift-left: w10 -> [w314]
    shift-right: [w313] -> _
    shift-left: w5 -> [w319]
    shift-right: [w318] -> _
    stop <- w312 continue-if-true
    # "Stop loop when exit button hit."
    n112 = stacked-sequence {
      seq-local: [_ _ _ _ w415 _ _ _ _ _ _ _] -> [_ _ _ _ _ w461 _ _ _ _ _ _]
      seq-local: [_ _ _ _ _ _ w508 _ _ _ _ _] -> [_ _ _ _ _ _ _ _ w568 _ _ _]
      seq-local: [_ _ _ _ _ _ _ _ w567 _ _ _] -> [_ _ _ _ _ _ _ _ _ w634 _ _]
      seq-local: [_ _ _ _ _ _ _ _ _ _ w650 _] -> [_ _ _ _ _ _ _ _ _ _ _ w705]
      seq-local: [_ _ _ _ _ w460 _ _ _ _ _ _] -> [_ _ _ _ _ _ w506 _ _ _ _ _]
      seq-local: [_ _ _ _ _ _ _ _ _ _ w649 _] -> [_ _ _ _ _ _ _ _ _ _ _ w703]
      seq-local: [w335 _ _ _ _ _ _ _ _ _ _ _] -> [_ w380 w392 w403 _ _ _ _ _ _ _ _]
      seq-local: [w332 _ _ _ _ _ _ _ _ _ _ _] -> [_ _ _ _ w416 _ _ _ _ _ _ _]
      seq-local: [w333 _ _ _ _ _ _ _ _ _ _ _] -> [_ w378 w389 w400 _ _ _ _ _ _ _ _]
      seq-local: [_ _ _ _ _ _ _ _ _ w631 _ _] -> [_ _ _ _ _ _ _ _ _ _ w648 _]
      seq-local: [_ _ _ _ w414 _ _ _ _ _ _ _] -> [_ _ _ _ _ _ _ _ w561 _ _ _]
      seq-local: [_ _ _ _ _ w458 _ _ _ _ _ _] -> [_ _ _ _ _ _ _ _ w560 _ _ _]
      seq-local: [_ _ _ _ _ _ w505 _ _ _ _ _] -> [_ _ _ _ _ _ _ _ w559 _ _ _]
      seq-local: [_ _ _ _ w411 _ _ _ _ _ _ _] -> [_ _ _ _ _ w456 _ _ _ _ _ _]
      seq-local: [_ _ _ _ _ w455 _ _ _ _ _ _] -> [_ _ _ _ _ _ w503 _ _ _ _ _]
      seq-local: [_ _ _ _ _ _ w502 _ _ _ _ _] -> [_ _ _ _ _ _ _ w548 w558 _ _ _]
      seq-local: [w331 _ _ _ _ _ _ _ _ _ _ _] -> [_ w377 w388 w399 _ _ _ _ _ _ _ _]
      seq-local: [_ _ _ _ _ _ _ _ w550 _ _ _] -> [_ _ _ _ _ _ _ _ _ _ w643 _]
      tunnel: w314 -> [w336 _ _ _ w419 w464 w511 _ w571 w636 w657 w694]
      tunnel: [_ _ _ _ _ _ _ _ w564 _ _ _] -> w318
      tunnel: w319 -> [_ w379 _ _ w417 _ _ _ w554 _ w653 w697]
      tunnel: w317 -> [_ _ w390 _ _ w459 _ _ w552 _ w652 w696]
      tunnel: w316 -> [_ _ _ w401 _ _ w507 _ w553 _ w651 w695]
      tunnel: [_ _ _ _ _ _ _ _ w562 _ _ _] -> w315
      tunnel: [_ _ _ _ _ _ _ _ _ _ w656 _] -> w313
      tunnel: [_ _ _ _ _ _ _ _ _ _ _ w692] -> w312
      tunnel: w306 -> [w334 w381 w391 w402 w418 w463 w510 _ w565 _ w654 w699]
      tunnel: w311 -> [w330 _ _ _ _ _ _ _ _ _ _ _]
      tunnel: [_ _ _ _ _ _ _ _ _ _ _ w693] -> w310
      tunnel: [_ _ _ _ _ _ _ _ w563 _ _ _] -> w309
      tunnel: w308 -> [_ _ _ _ w412 w457 w504 _ w569 _ w645 _]
      tunnel: [_ _ _ _ _ _ _ _ w570 _ _ _] -> w307
      tunnel: [_ _ _ _ _ _ _ _ _ _ w655 _] -> w305
      tunnel: w304 -> [_ _ _ _ _ _ _ _ w555 w630 _ w698]
      tunnel: [_ _ _ _ _ _ _ _ _ w632 _ _] -> w303
      tunnel: w302 -> [_ _ _ _ w410 w454 w501 _ w551 _ _ _]
      tunnel: [_ _ _ _ _ _ _ _ _ _ w644 _] -> w301
      tunnel: w300 -> [w320 _ _ _ _ _ _ _ _ _ _ _]
      tunnel: [w327 _ _ _ _ _ _ _ _ _ _ _] -> w299
      tunnel: [w329 _ _ _ _ _ _ _ _ _ _ _] -> w298
      tunnel: w297 -> [w328 _ _ _ _ _ _ _ _ _ _ _]
      tunnel: w296 -> [w326 _ _ _ _ _ _ _ _ _ _ _]
      tunnel: w295 -> [w325 _ _ _ _ _ _ _ _ _ _ _]
      frame #0 {
        n113 = Tick Count (ms)() -> (millisecond timer value=w322:u32)
        n114 = Add(x=w320, y="SAMPLE TIME, ms") -> (x+y=w321:u32)
        n115 = Greater Or Equal?(x=w322, y=w321) -> (x >= y?=w323:bool)
        n116 = case shown="真" w323 {
          tunnel: [FALSE w372] -> w331
          tunnel: [w340 w364] -> w332
          tunnel: [w342 w363] -> w333
          tunnel: w334 -> [w343 w362]
          tunnel: [w338 w359] -> w335
          tunnel: w330 -> [w341 w360]
          tunnel: w336 -> [_ w361]
          tunnel: [w338 w359] -> w329
          tunnel: w328 -> [w338 _]
          tunnel: w322 -> [_ w349]
          tunnel: [w337 w348] -> w327
          tunnel: w320 -> [w337 _]
          tunnel: w321 -> [_ w348]
          tunnel: w326 -> [_ w355]
          tunnel: w325 -> [_ w356]
          frame False {
            n117 = call "Get elapsed time.vi"("Pump? (F:pump present)."=w343, "Error in (no error)."=w341) -> ("Duration of run\n(Hours:minutes:seconds."=w342:T19, "Error out."=w340:errorcluster)  [unwired: 1 out]
          }
          frame True {
            w353 = "="
            # "Error cluster."
            # "Get flow rate, pressure, volume, operation status, control status, problem status, analog input Voltages, digital input string, multipump data and timing info."
            # "Bad checksum?"
            n118 = Subtract(x=w349, y=w356) -> (x-y=w347:u32)
            "TOTAL TIME, ms" <- w347
            n119 = Number To Decimal String(number=w347) -> (decimal integer string=w352:string)  [unwired: 1 in]
            n120 = call "Get all pump data.vi"("Port/Baud/Controller"=w361, "Error in (no error)."=w360) -> ("Reply string."=w354:string, "Status of the data."=w371:T20)  [unwired: 1 out]
            n121 = Unbundle By Name(w371) -> ("Bad checksum?"=w372:bool)
            n122 = Match True/False String(2:w353, 3:w353, 4:w354) -> (1:w350:string)  [unwired: 1 out]
            n123 = Concatenate Strings(w352, ",", w350, "\r", "\n") -> (w345:string)
            n124 = call "Get elapsed time.vi"("Pump? (F:pump present)."=w362) -> ("Duration of run\n(Hours:minutes:seconds."=w363:T19, "Error out."=w365:errorcluster)  [unwired: 1 in, 1 out]
            n125 = case shown="真" "?" {
              tunnel: w345 -> [_ w376]
              tunnel: w355 -> [_ w375]
              frame False {
              }
              frame True {
                n126 = call <vilib>:"Write Characters To File.vi"("append to file? (new file:F)"=TRUE, "character string"=w376, "file path (dialog if empty)"=w375) -> ()  [unwired: 2 in, 1 out]
              }
            }
            n127 = call "Parse Get All reply string (3 pumps).vi"("Reply string (empty)."=w354, "Error in (no error)."=w365) -> ("Data."=w359:T21, "Pump status."=→"Pump status.":T1, "Error out."=w369:errorcluster)
            n128 = call "Parse analog Voltages.vi"("Error in (no error)."=w369, "Reply string (empty)."=w354) -> ("Error out."=w367:errorcluster, "Analog input Voltages."=→"Analog input Voltages.":T22)
            n129 = call "Parse digital inputs.vi"("Reply string (empty)."=w354, "Error in (no error)."=w367) -> ("Digital input string."=→"Digital input string.":string, "Error out."=w370:errorcluster)  [unwired: 2 in]
            n130 = call "Parse multipump outputs.vi"("Reply string (empty)."=w354, "Error in (no error)."=w370) -> ("Multipump data."=→"Multipump data.":T2, "Error out."=w364:errorcluster)  [unwired: 2 in]
          }
        }
      }
      frame #1 {
        # "Display data and status info for pump A."
        # "Bad checksum?"
        n131 = case shown="假" w377 {
          tunnel: w378 -> [w387 _]
          tunnel: w379 -> [w385 _]
          tunnel: w380 -> [w383 _]
          tunnel: w381 -> [w382 _]
          frame False {
            w386 = u8 0  # Pump A.
            n132 = call "Display data.vi"("Pump? (F:pump present)."=w382, "Pump Settings"=w385, "Pump (0:A)."=w386, "Duration of run\n(Hours:minutes:seconds."=w387, "Data."=w383) -> ("Pump output."=→"Pump A output.":T8)  [unwired: 2 in]
          }
          frame True {
            # "Checksum invalid; do not update display."
          }
        }
      }
      frame #2 {
        # "Display data and status info for pump B."
        # "Bad checksum?"
        n133 = case shown="假" w388 {
          tunnel: w389 -> [w397 _]
          tunnel: w390 -> [w396 _]
          tunnel: w391 -> [w395 _]
          tunnel: w392 -> [w394 _]
          frame False {
            w398 = u8 1  # Pump B.
            n134 = call "Display data.vi"("Pump? (F:pump present)."=w395, "Pump Settings"=w396, "Pump (0:A)."=w398, "Duration of run\n(Hours:minutes:seconds."=w397, "Data."=w394) -> ("Pump output."=→"Pump B output.":T8)  [unwired: 2 in]
          }
          frame True {
            # "Checksum invalid; do not update display."
          }
        }
      }
      frame #3 {
        # "Display data and status info for pump B."
        # "Bad checksum?"
        n135 = case shown="假" w399 {
          tunnel: w400 -> [w409 _]
          tunnel: w401 -> [w407 _]
          tunnel: w402 -> [w406 _]
          tunnel: w403 -> [w405 _]
          frame False {
            w408 = u8 2  # Pump C.
            n136 = call "Display data.vi"("Pump? (F:pump present)."=w406, "Pump Settings"=w407, "Pump (0:A)."=w408, "Duration of run\n(Hours:minutes:seconds."=w409, "Data."=w405) -> ("Pump output."=→"Pump C output.":T8)  [unwired: 2 in]
          }
          frame True {
            # "Checksum invalid; do not update display."
          }
        }
      }
      frame #4 {
        # "Check for a change in pump A settings.  If so, switch to REMOTE and write changes to pump controller"
        # "Error cluster out."
        n137 = Unbundle(w418) -> (w413:bool)  [unwired: 2 out]
        n138 = case shown="假" w413 {
          tunnel: w419 -> [w429 _]
          tunnel: w416 -> [w423 w453]
          tunnel: [w428 w453] -> w415
          tunnel: w417 -> [w426 w452]
          tunnel: [w425 w452] -> w414
          tunnel: w412 -> [w422 _]
          tunnel: [w421 FALSE] -> w411
          tunnel: w410 -> [w420 _]
          frame False {
            # "Error cluster in."
            n139 = Not Equal?(x="Pump A Settings", y=w426) -> (x != y?=w427:bool)
            n140 = case shown="假" w427 {
              selector: w427 -> [w430 _]
              tunnel: w423 -> [w432 w438]
              tunnel: w429 -> [_ w441]
              tunnel: [w432 w444] -> w428
              tunnel: w426 -> [w431 w440]
              tunnel: [w431 w443] -> w425
              tunnel: "Pump A Settings" -> [_ w442]
              tunnel: w422 -> [_ w437]
              tunnel: [w430 w435] -> w421
              tunnel: w420 -> [_ w433]
              frame False {
                # "Old Pump A Settings"
              }
              frame True {
                w434 = u8 0  # Pump A
                n141 = Equal To 0?(x=w437) -> (x = 0?=w436:bool)
                n142 = case shown="假" w436 {
                  tunnel: w441 -> [w448 _]
                  tunnel: w438 -> [w447 w450]
                  tunnel: [w446 w450] -> w439
                  tunnel: [TRUE FALSE] -> w435
                  frame False {
                    n143 = call "Remote/local.vi"("Error in (no error)."=w447, "Port/Baud/Controller"=w448) -> ("Error out."=w446:errorcluster)  [unwired: 3 in]
                  }
                  frame True {
                  }
                }
                n144 = call "Single pump operations.vi"("Old pump Settings."=w440, "New pump Settings."=w442, "Error in (no error)."=w439, "Pump (0:A)."=w434, "Physical and alarm limits"=w433, "Port/Baud/Controller"=w441) -> ("Error out."=w444:errorcluster, "New pump Settings."=w443:T6)
                n145 = local write "Pump A Settings"(w443) -> ()
              }
            }
          }
          frame True {
          }
        }
      }
      frame #5 {
        # "Check for a change in pump B settings.  If so, switch to REMOTE and write changes to pump controller"
        # "Error cluster out."
        n146 = Unbundle(w463) -> (w462:bool)  [unwired: 2 out]
        n147 = case shown="假" w462 {
          tunnel: w464 -> [w470 _]
          tunnel: w461 -> [w469 w499]
          tunnel: [w475 w499] -> w460
          tunnel: w459 -> [w473 w500]
          tunnel: [w471 w500] -> w458
          tunnel: w457 -> [w468 _]
          tunnel: [w467 w498] -> w455
          tunnel: w456 -> [w466 w498]
          tunnel: w454 -> [w465 _]
          frame False {
            # "Error cluster in."
            n148 = Not Equal?(x="Pump B Settings", y=w473) -> (x != y?=w474:bool)
            n149 = case shown="假" w474 {
              tunnel: [w477 w491] -> w475
              tunnel: w473 -> [w478 w490]
              tunnel: "Pump B Settings" -> [_ w488]
              tunnel: [w478 w489] -> w471
              tunnel: w470 -> [_ w486]
              tunnel: w469 -> [w477 w485]
              tunnel: w468 -> [_ w483]
              tunnel: [w476 w482] -> w467
              tunnel: w466 -> [w476 w481]
              tunnel: w465 -> [_ w480]
              frame False {
                # "Old Pump A Settings"
              }
              frame True {
                w479 = u8 1  # Pump B
                n150 = Equal To 0?(x=w483) -> (x = 0?=w487:bool)
                n151 = case shown="假" w487 {
                  tunnel: w486 -> [w495 _]
                  tunnel: w485 -> [w494 w497]
                  tunnel: [w493 w497] -> w484
                  tunnel: [TRUE w496] -> w482
                  tunnel: w481 -> [_ w496]
                  frame False {
                    n152 = call "Remote/local.vi"("Error in (no error)."=w494, "Port/Baud/Controller"=w495) -> ("Error out."=w493:errorcluster)  [unwired: 3 in]
                  }
                  frame True {
                  }
                }
                n153 = call "Single pump operations.vi"("Old pump Settings."=w490, "New pump Settings."=w488, "Error in (no error)."=w484, "Pump (0:A)."=w479, "Physical and alarm limits"=w480, "Port/Baud/Controller"=w486) -> ("Error out."=w491:errorcluster, "New pump Settings."=w489:T6)
                n154 = local write "Pump B Settings"(w489) -> ()
              }
            }
          }
          frame True {
          }
        }
      }
      frame #6 {
        # "Check for a change in pump C settings.  If so, switch to REMOTE and write changes to pump controller"
        # "Error cluster out."
        n155 = Unbundle(w510) -> (w509:bool)  [unwired: 2 out]
        n156 = case shown="假" w509 {
          tunnel: w511 -> [w517 _]
          tunnel: [w522 w547] -> w508
          tunnel: w507 -> [w520 w546]
          tunnel: w506 -> [w516 w547]
          tunnel: [w518 w546] -> w505
          tunnel: w504 -> [w515 _]
          tunnel: w503 -> [w513 w545]
          tunnel: [w514 w545] -> w502
          tunnel: w501 -> [w512 _]
          frame False {
            # "Error cluster in."
            n157 = Not Equal?(x="Pump C Settings", y=w520) -> (x != y?=w521:bool)
            n158 = case shown="假" w521 {
              tunnel: [w524 w538] -> w522
              tunnel: w520 -> [w525 w537]
              tunnel: "Pump C Settings" -> [_ w535]
              tunnel: [w525 w536] -> w518
              tunnel: w517 -> [_ w533]
              tunnel: w516 -> [w524 w532]
              tunnel: w515 -> [_ w531]
              tunnel: [w523 w529] -> w514
              tunnel: w513 -> [w523 w528]
              tunnel: w512 -> [_ w527]
              frame False {
                # "Old Pump A Settings"
              }
              frame True {
                w526 = u8 2  # Pump C
                n159 = Equal To 0?(x=w531) -> (x = 0?=w534:bool)
                n160 = case shown="假" w534 {
                  tunnel: w533 -> [w542 _]
                  tunnel: w532 -> [w541 w544]
                  tunnel: [w540 w544] -> w530
                  tunnel: [TRUE w543] -> w529
                  tunnel: w528 -> [_ w543]
                  frame False {
                    n161 = call "Remote/local.vi"("Error in (no error)."=w541, "Port/Baud/Controller"=w542) -> ("Error out."=w540:errorcluster)  [unwired: 3 in]
                  }
                  frame True {
                  }
                }
                n162 = call "Single pump operations.vi"("Old pump Settings."=w537, "New pump Settings."=w535, "Error in (no error)."=w530, "Pump (0:A)."=w526, "Physical and alarm limits"=w527, "Port/Baud/Controller"=w533) -> ("Error out."=w538:errorcluster, "New pump Settings."=w536:T6)
                n163 = local write "Pump C Settings"(w536) -> ()
              }
            }
          }
          frame True {
          }
        }
      }
      frame #7 {
        # "If in LOCAL and the user changed a front panel setting switch to REMOTE and write changes to pump controller in fram 4, 5, or 6 depending on the pump.  Here reset the indicator on the front panel to show we are in REMOTE."
        n164 = case shown="真" w548 {
          frame False {
          }
          frame True {
            n165 = local write "Remote/Local/External (0:Remote)."(0) -> ()
          }
        }
      }
      frame #8 {
        # "Check for a change in the REMOTE/LOCAL/EXTERNAL control and write any changes to the pump controller."
        n166 = Equal?(x="Remote/Local/External (0:Remote).", y=w569) -> (x = y?=w557:bool)
        n167 = Or(x=w558, y=w557) -> (x .or. y?=w556:bool)
        n168 = case shown="假" w556 {
          tunnel: [w588 w628] -> w567
          tunnel: "Remote/Local/External (0:Remote)." -> [w574 _]
          tunnel: w571 -> [w587 _]
          tunnel: w569 -> [_ w629]
          tunnel: [w574 w629] -> w570
          tunnel: w568 -> [w586 w628]
          tunnel: w565 -> [w585 _]
          tunnel: [w584 w627] -> w564
          tunnel: [w583 w626] -> w563
          tunnel: [w582 w625] -> w562
          tunnel: w561 -> [w581 w627]
          tunnel: w560 -> [w580 w626]
          tunnel: w559 -> [w579 w625]
          tunnel: w555 -> [w578 _]
          tunnel: w554 -> [w577 _]
          tunnel: w553 -> [w576 _]
          tunnel: w552 -> [w575 _]
          tunnel: w551 -> [w573 w624]
          tunnel: [w572 w624] -> w550
          frame False {
            n169 = case "Case" shown="\"EXTERNAL\"" w574 {
              tunnel: w586 -> [w610 w618 w619]
              tunnel: w587 -> [w595 w617 _]
              tunnel: [w592 w616 w619] -> w588
              tunnel: w585 -> [w594 _ _]
              tunnel: [w604 w614 w620] -> w584
              tunnel: [w603 w613 w621] -> w583
              tunnel: [w602 w612 w622] -> w582
              tunnel: w581 -> [_ w614 w620]
              tunnel: w580 -> [_ w613 w621]
              tunnel: w579 -> [_ w612 w622]
              tunnel: w578 -> [w600 _ _]
              tunnel: w577 -> [w599 _ _]
              tunnel: w576 -> [w597 _ _]
              tunnel: w575 -> [w598 _ _]
              tunnel: w573 -> [w590 w611 w623]
              tunnel: [w589 w611 w623] -> w572
              frame "REMOTE" {
                n170 = call "Remote/local.vi"("Error in (no error)."=w610, "REMOTE/LOCAL (F:REMOTE)."=FALSE, "Port/Baud/Controller"=w595) -> ("Error out."=w601:errorcluster)  [unwired: 2 in]
                n171 = Build Array(w599, w598, w597) -> (w596:T11)
                n172 = call "Setup remote.vi"("Port/Baud/Controller"=w595, "Array of pump settings."=w596, "Pump? (F:pump present)."=w594, "Mode (0:INDEPENDENT)."=w600, "Error in (no error)."=w601) -> ("Array of pump settings."=w605:T11, "Error out."=w593:errorcluster)  [unwired: 2 in]
                n173 = Index Array(array=w605, index=2) -> (element=w602:T6)
                n174 = call "Update alarm limits.vi"("Error in (no error)."=w593, "Pump? (F:pump present)."=w594, "Port/Baud/Controller"=w595) -> ("Error out."=w592:errorcluster, "Alarm limits setpoints (psi and ml/min)."=w591:T23)
                n175 = local write "Pump C Settings"(w602) -> ()
                n176 = Index Array(array=w605, index=0) -> (element=w604:T6)
                n177 = Index Array(array=w605, index=1) -> (element=w603:T6)
                n178 = local write "Pump B Settings"(w603) -> ()
                n179 = local write "Pump A Settings"(w604) -> ()
                n180 = Bundle(cluster=w590, w591) -> (w589:T17)  [unwired: 1 in]
              }
              frame "LOCAL" {
                n181 = call "Remote/local.vi"("Error in (no error)."=w618, "REMOTE/LOCAL (F:REMOTE)."=TRUE, "Port/Baud/Controller"=w617) -> ("Error out."=w616:errorcluster)  [unwired: 2 in]
              }
              frame "EXTERNAL" {
              }
            }
          }
          frame True {
          }
        }
      }
      frame #9 {
        # "Check for a change in the INDEPENDENT/multipump control on the front panel and write any changes to the pump controller."
        # "Execute Menu Buttons"
        n182 = Equal?(x="Control mode (0:INDEPENDENT).", y=w630) -> (x = y?=w635:bool)
        n183 = case shown="假" w635 {
          tunnel: [w640 w641] -> w631
          tunnel: "Control mode (0:INDEPENDENT)." -> [w637 _]
          tunnel: w636 -> [w639 _]
          tunnel: w630 -> [_ w642]
          tunnel: [w637 w642] -> w632
          tunnel: w634 -> [w638 w641]
          frame False {
            n184 = call "Set controller mode.vi"("Error in (no error)."=w638, "Mode (0:INDEPENDENT)."=w637, "Port/Baud/Controller"=w639) -> ("Error out."=w640:errorcluster)  [unwired: 2 in]
          }
          frame True {
          }
        }
      }
      frame #10 {
        # "Check if one of the keys on the tool bar on the front panel has been clicked.  If so, do what ever action the key is wired to."
        # "Quit?"
        # "Error cluster."
        # "Execute Menu Buttons"
        n185 = Cluster To Array(cluster="Tasks.") -> (array=w660:bool[])
        n186 = call "Which Button.vi"("Menu Buttons"=w660) -> ("Index"=w658:i32)
        n187 = Type Cast(type=T18."Quit", x=w658) -> (*(type *) &x=w647:T18)
        n188 = case shown="\"Reconfigure\"" w647 {
          tunnel: [w664 w676 w685 w690] -> w656
          tunnel: w657 -> [w664 w672 w685 w690]
          tunnel: [TRUE TRUE TRUE FALSE] -> w650
          tunnel: [w663 w677 w683 w689] -> w655
          tunnel: w648 -> [w662 w673 w682 w688]
          tunnel: [w662 w674 w684 w688] -> w649
          tunnel: w654 -> [w663 w677 w683 w689]
          tunnel: w653 -> [_ _ _ _]
          tunnel: w652 -> [_ _ _ _]
          tunnel: w651 -> [_ _ _ _]
          tunnel: w645 -> [_ w675 _ _]
          tunnel: [w661 w671 w680 w687] -> w644
          tunnel: w643 -> [w661 w671 w679 w687]
          frame "No op" {
          }
          frame "Reconfigure" {
            # "Path to serial port config file."
            n189 = call <vilib>:"Application Directory.vi"() -> ("Application Directory"=w669:path)
            n190 = Path To String(path=w669) -> (string=w668:string)
            n191 = Concatenate Strings(w668, "\\data\\Config.prt" ("字符串")) -> (w670:string)
            n192 = String To Path(string=w670) -> (path=w666:path)
            n193 = call "Reconfigure.vi"("Error in (no error)."=w673, "Remote/Local/External (0:Remote)."=w675, "Serial port config file (empty)."=w666, "Port/Baud/Controller"=w672) -> ("Error out."=w674:errorcluster, "Port/Baud/Controller"=w676:T10)  [unwired: 1 in]
          }
          frame "alarm limits" {
            n194 = call "Alarm Limits.vi"("Error in (no error)."=w682, "Pump? (F:pump present)."=w683, "Port/Baud/Controller"=w685) -> ("Error out."=w684:errorcluster, "Alarm limits setpoints (psi and ml/min)."=w681:T23)  [unwired: 1 in]
            n195 = Bundle(cluster=w679, w681) -> (w680:T17)  [unwired: 1 in]
          }
          frame "Quit" {
          }
        }
      }
      frame #11 {
        # "Stop on an error or if the QUIT key has been clicked."
        # "Error cluster."
        # "Quit?"
        n196 = Unbundle By Name(w703) -> ("code"=w702:i32)
        n197 = Equal?(x=1, y=w702) -> (x = y?=w700:bool)
        n198 = case shown="假" w700 {
          tunnel: w703 -> [w709 _]
          tunnel: [w708 w710] -> w693
          tunnel: [w707 TRUE] -> w704
          frame False {
            n199 = call <vilib>:"General Error Handler.vi"("error in (no error)"=w709) -> ("error?"=w706:bool, "error out"=w708:errorcluster)  [unwired: 10 in, 3 out]
            n200 = Not(x=w706) -> (.not. x?=w707:bool)
          }
          frame True {
            n201 = call <vilib>:"Simple Error Handler.vi"() -> ("error out"=w710:errorcluster)  [unwired: 5 in, 4 out]
          }
        }
        n202 = And(x=w704, y=w705) -> (x .and. y?=w692:bool)
        n203 = case shown="真" w692 {
          tunnel: w694 -> [w719 _]
          tunnel: w698 -> [w717 _]
          tunnel: w699 -> [w716 _]
          tunnel: w697 -> [w715 _]
          tunnel: w696 -> [w714 _]
          tunnel: w695 -> [w713 _]
          frame False {
            n204 = Current VI's Path() -> (path=w720:path)
            n205 = Build Array(w715, w714, w713) -> (w712:T11)
            n206 = Strip Path(path=w720) -> (stripped path=w722:path)  [unwired: 1 out]
            n207 = Build Path(base path=w722, name or relative path="Config.prt") -> (appended path=w718:path)
            n208 = call "Quit.vi"("Port/Baud/Controller"=w719, "Pump? (F:pump present)."=w716, "Serial port config file (empty)."=w718, "Mode (0:INDEPENDENT)."=w717, "Array of pump settings."=w712) -> ()  [unwired: 3 in, 1 out]
          }
          frame True {
          }
        }
      }
    }
  }
